vi "Analog Input - 1 Channel - Continuous Sampling.vi"() -> ()   [LabVIEW 2019]
uses:
  <vilib>/myRIO/Instrument Drivers/Onboard IO/AI Continuous/typedefs/AI Continuous Reference.ctl
  <vilib>/myRIO/Common/Instrument Driver Framework/Utilities/typedefs/myRIO Generic Hardware Reference.ctl
  <vilib>/myRIO/Common/Instrument Driver Framework/Utilities/typedefs/Hardware Version Enum.ctl
  <vilib>/myRIO/Common/Instrument Driver Framework/Utilities/typedefs/myRIO v1.0 Reference.ctl
  <vilib>/myRIO/Common/Instrument Driver Framework/Utilities/typedefs/Generic FPGA Reference.ctl
  <vilib>/myRIO/Common/Instrument Driver Framework/ELVIS III v1.0/AI Continuous/typedefs/AI Continuous Channels List.ctl
  <vilib>/myRIO/Common/Instrument Driver Framework/ELVIS III v1.0/AI Continuous/typedefs/ELVIS III v1.0 AI Continuous Channels Enum.ctl
  <vilib>/myRIO/Common/Instrument Driver Framework/Utilities/typedefs/Analog Scaling Constants.ctl
  <vilib>/userdefined/High Color/nirio_resource_hc.ctl
  <vilib>/myRIO/Common/Instrument Driver Framework/ELVIS III v1.0/AI Continuous/vis/ELVIS III v1.1 Open AI (Continuous).vi
  <vilib>/myRIO/Common/Instrument Driver Framework/Utilities/vis/Validate Channels.vi
  <vilib>/myRIO/Common/Instrument Driver Framework/ELVIS III v1.0/AI Continuous/vis/ELVIS III v1.0 Reserve AI Continuous.vi
  <vilib>/myRIO/Common/Instrument Driver Framework/ELVIS III v1.0/AI Continuous/vis/ELVIS III v1.0 Close AI Continuous.vi
  <vilib>/myRIO/Common/Instrument Driver Framework/myRIO v1.0/UART/vis/myRIO v1.0 Close UART.vi
  <vilib>/myRIO/Common/Instrument Driver Framework/ELVIS III v1.0/AI Continuous/vis/ELVIS III v1.0 Build MUX Configuration AI Continuous.vi
  <vilib>/myRIO/Common/Instrument Driver Framework/ELVIS III v1.0/AI Continuous/vis/ELVIS III v1.0 Unreserve AI Continuous.vi
  <vilib>/Utility/VariantDataType/GetNumericInfo.vi
  <vilib>/Utility/error.llb/Error Cluster From Error Code.vi
  <vilib>/myRIO/Common/Instrument Driver Framework/ELVIS III v1.0/ELVIS III v1.1 Open.vi
  <vilib>/myRIO/Common/Instrument Driver Framework/ELVIS III v1.0/Resource Manager/vis/ELVIS III v1.0 Coerce AI Scaling.vi
  <vilib>/myRIO/Common/Instrument Driver Framework/ELVIS III v1.0/Resource Manager/vis/ELVIS III v1.0 Reserve Channel List.vi
  <vilib>/myRIO/Common/Instrument Driver Framework/ELVIS III v1.0/Resource Manager/vis/ELVIS III v1.0 Configure DMAs.vi
  <vilib>/myRIO/Common/Instrument Driver Framework/myRIO v1.0/myRIO v1.0 Close.vi
  <vilib>/myRIO/Common/Instrument Driver Framework/ELVIS III v1.0/AI Continuous/vis/ELVIS III v1.1 Stop AI Continuous.vi
  <vilib>/myRIO/Common/Instrument Driver Framework/ELVIS III v1.0/AI Continuous/vis/ELVIS III v1.1 Start AI Continuous.vi
  <vilib>/myRIO/Common/Instrument Driver Framework/ELVIS III v1.0/AI Continuous/vis/ELVIS III v1.0 AI Continuous Read.vi
  <vilib>/myRIO/Common/Instrument Driver Framework/ELVIS III v1.0/Resource Manager/vis/ELVIS III v1.0 Unreserve Channel List.vi
  <vilib>/myRIO/Common/Instrument Driver Framework/Utilities/vis/FPGA Ref Manager.vi
  <vilib>/myRIO/Common/Instrument Driver Framework/ELVIS III v1.0/ELVIS III v1.0 Reset FPGA.vi
  <vilib>/myRIO/Common/Instrument Driver Framework/myRIO v1.0/IRQ/vis/myRIO v1.0 IRQ Info FGV.vi
  <vilib>/myRIO/Common/Instrument Driver Framework/myRIO v1.0/IRQ/vis/myRIO v1.0 Timer IRQ Info FGV.vi
  <vilib>/myRIO/Common/Instrument Driver Framework/myRIO v1.0/IRQ/vis/myRIO v1.0 ISR Agent.vi
  <vilib>/myRIO/Instrument Drivers/Utilities/vis/Reset Index.vi
  <vilib>/myRIO/Common/Instrument Driver Framework/myRIO v1.0/Resource Manager/vis/myRIO v1.0 Block Write Resource Manager.vi
  <vilib>/myRIO/Instrument Drivers/Onboard IO/AI Continuous/vis/myRIO AI Continuous Open.xnode
  <vilib>/myRIO/Instrument Drivers/Utilities/Utilities.lvlib
  <vilib>/myRIO/Instrument Drivers/Onboard IO/AI Continuous/AI Continuous.lvlib
panel:
  out "Analog Data":dbl[](graph)
  in  "Stop":bool
  # "ELVIS III Control IO"
  # "模拟输入单通道"
  # "Overview: Acquires voltage values continuously from Bank A, Channel 0 (A/AI0) until the acquisition is stopped.\nInstructions:\n1. Connect A/AI0 to a valid signal.\n2. Run the VI."
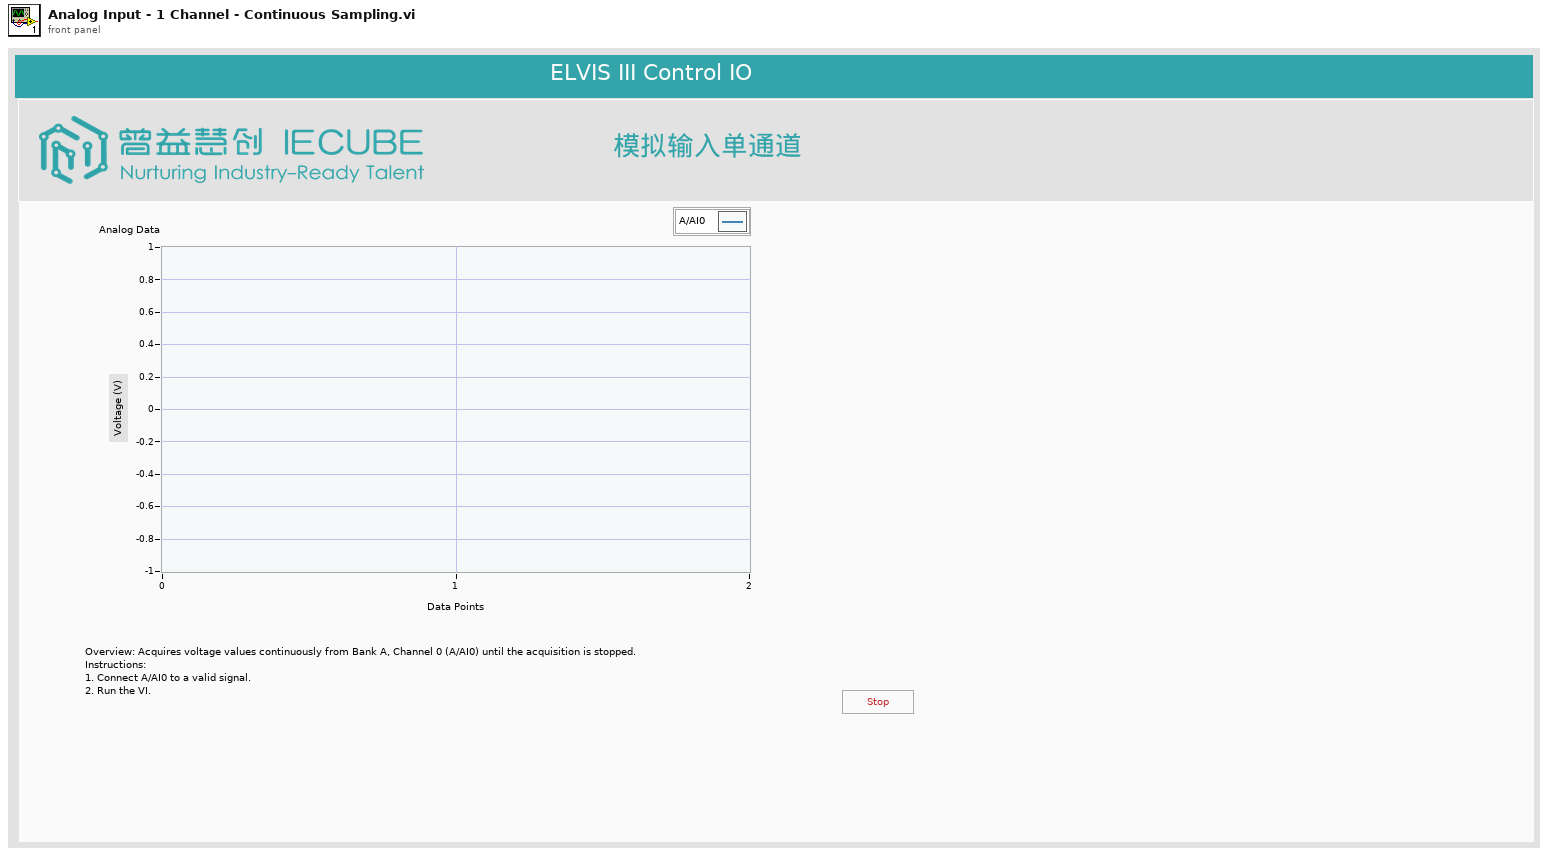
[diagram p1: front panel]
types:
  T1 = typedef "nirio_resource_hc.ctl" = tag
  T2 = typedef "Hardware Version Enum.ctl" = enum16{"Unknown", "myRIO-1900", "myRIO-1950", "roboRIO", "NI ELVIS RIO CM", "ELVIS III"}
  T3 = typedef "AI Continuous.lvlib/AI Continuous Reference.ctl" = cluster{"myRIO Reference":T4, "AI (Continuous) Channels List":T7, "AI (Continuous) Scaling Constants List":T9[], "Bank Count":u8[]}
  T4 = typedef "myRIO Generic Hardware Reference.ctl" = cluster{"myRIO Model":T2, "myRIO Hardware Reference":T5}
  T5 = typedef "myRIO v1.0 Reference.ctl" = cluster{"Generic FPGA Reference":T6, "Allow multiple opens":bool}
  T6 = typedef "Generic FPGA Reference.ctl" = refnum<k20>
  T7 = typedef "AI Continuous Channels List.ctl" = T8[]
  T8 = typedef "ELVIS III v1.0 AI Continuous Channels Enum.ctl" = enum16{"Not Connected", "A/AI0 (Continuous)", "A/AI1 (Continuous)", "A/AI2 (Continuous)", "A/AI3 (Continuous)", "A/AI4 (Continuous)", "A/AI5 (Continuous)", "A/AI6 (Continuous)", "A/AI7 (Continuous)", "A/AI0 (DIFF Continuous)", "A/AI1 (DIFF Continuous)", "A/AI2 (DIFF Continuous)", "A/AI3 (DIFF Continuous)", "B/AI0 (Continuous)", "B/AI1 (Continuous)", "B/AI2 (Continuous)", "B/AI3 (Continuous)", "B/AI4 (Continuous)", "B/AI5 (Continuous)", "B/AI6 (Continuous)", "B/AI7 (Continuous)", "B/AI0 (DIFF Continuous)", "B/AI1 (DIFF Continuous)", "B/AI2 (DIFF Continuous)", "B/AI3 (DIFF Continuous)"}
  T9 = typedef "Analog Scaling Constants.ctl" = cluster{"LSB Weight (Volts)":dbl, "Offset (Volts)":dbl, "Signed?":bool}
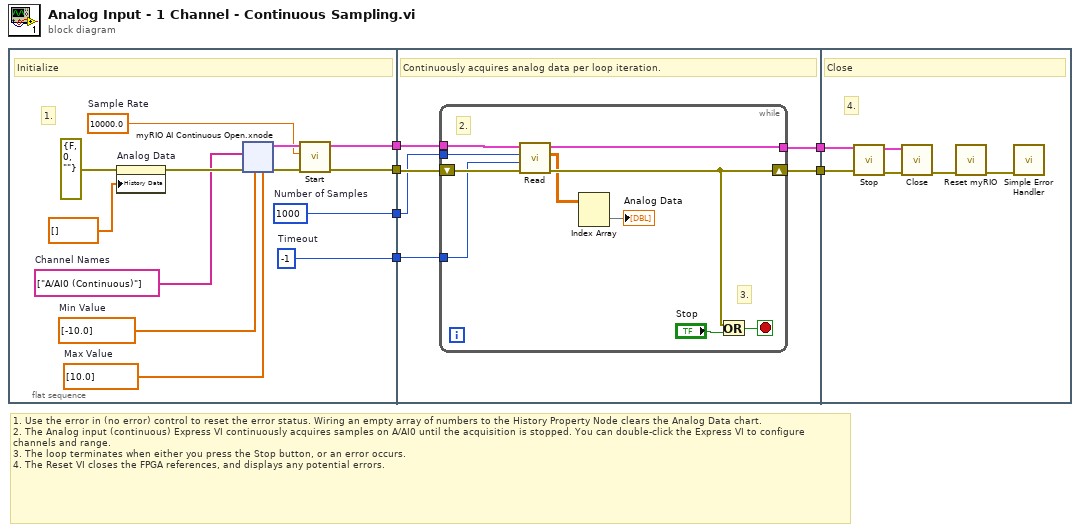
[diagram p0: block diagram]
diagram:
  # "1. Use the error in (no error) control to reset the error status. Wiring an empty array of numbers to the History Property Node clears the Analog Data chart.\n2. The Analog input (continuous) Express VI continuously acquires samples on A/AI0 until the acquisition is stopped. You can double-click the Express VI to configure channels and range.\n3. The loop terminates when either you press the Stop button, or an error occurs.\n4. The Reset VI closes the FPGA references, and displays any potential errors."
  n1 = flat-sequence {
    tunnel: [w14] -> w5
    tunnel: [w10] -> w4
    tunnel: [w8] -> w3
    tunnel: [w7] -> w2
    tunnel: [w46] -> w6
    tunnel: w5 -> [w45]
    tunnel: w4 -> [w42]
    tunnel: w3 -> [w43]
    tunnel: w2 -> [w44]
    tunnel: [w41] -> w1
    tunnel: w6 -> [w61]
    tunnel: w1 -> [w60]
    frame #0 {
      w8 = -1  # Timeout
      w7 = u32 1000  # Number of Samples
      w9 = 10000.0  # Sample Rate
      w11 = dbl[] [10.0]  # Max Value
      w12 = dbl[] [-10.0]  # Min Value
      w13 = tag[] ["A/AI0 (Continuous)"]  # Channel Names
      # "1."
      # "Initialize"
      n2 = property on="Analog Data" class="WFChart (严格)"(error in=errorcluster {"status"=FALSE, "code"=0, "source"=""} ("error constant"), "History Data"=dbl[] []) -> (error out=w15:errorcluster)  [unwired: 1 in, 1 out]
      n3 = xnode "myRIO AI Continuous Open.xnode"("error in (no error)"=w15, "Channel Names"=w13, "Max Value"=w11, "Min Value"=w12) -> ("error out"=w17:errorcluster, "AI (Continuous) Ref Out"=w16:T3)
      n4 = call <vilib>:"Start.vi"("error in (no error)"=w17, "Sample Rate"=w9, "AI (Continuous) Ref In"=w16) -> ("error out"=w14:errorcluster, "AI (Continuous) Ref Out"=w10:T3)  [unwired: 7 in]
    }
    frame #1 {
      # "Continuously acquires analog data per loop iteration."
      n5 = while {
        shift-right: [w53] -> w46
        shift-left: w45 -> [w54]
        tunnel: w44 -> [w52]
        tunnel: w43 -> [w51]
        tunnel: w42 -> [w50]
        tunnel: [w47] -> w41
        stop <- w55 stop-if-true
        # "3."
        # "2."
        n6 = call <vilib>:"Read.vi"("error in (no error)"=w54, "Timeout"=w51, "Number of Samples"=w52, "AI (Continuous) Ref In"=w50) -> ("error out"=w53:errorcluster, "Values"=w49:dbl[][], "AI (Continuous) Ref Out"=w47:T3)  [unwired: 5 in]
        n7 = Index Array(array=w49) -> (element=→"Analog Data":dbl[])  [unwired: 2 in]
        n8 = Or(x=w53, y="Stop") -> (x .or. y?=w55:bool)
      }
    }
    frame #2 {
      # "4."
      # "Close"
      n9 = call <vilib>:"Stop.vi"("error in (no error)"=w61, "AI (Continuous) Ref In"=w60) -> ("error out"=w58:errorcluster, "AI (Continuous) Ref Out"=w59:T3)  [unwired: 8 in]
      n10 = call <vilib>:"Close.vi"("error in (no error)"=w58, "AI (Continuous) Ref In"=w59) -> ("error out"=w57:errorcluster)  [unwired: 9 in]
      n11 = call <vilib>:"Reset myRIO.vi"("error in (no error)"=w57) -> ("error out"=w62:errorcluster)  [unwired: 10 in]
      n12 = call <vilib>:"Simple Error Handler.vi"("error in (no error)"=w62) -> ()  [unwired: 4 in, 5 out]
    }
  }
